vi "medir temp.vi"(2 "multimetro":u16(ring) items=["3458", "34420", "34401"], 3 "Medir Temperatura":bool, 4 "address string":string) -> (1 "Numeric":ext)   [LabVIEW 2014]
uses:
  <vilib>/Analysis/NI_AALBase.lvlib
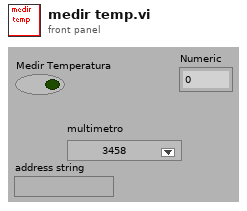
[diagram p1: front panel]
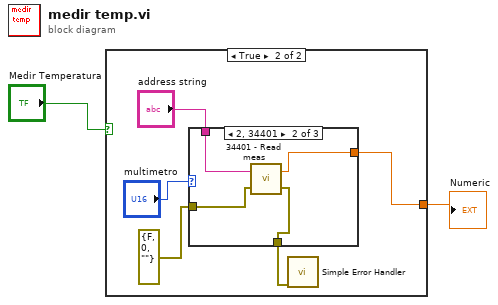
[diagram p0: block diagram]
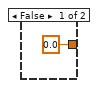
[diagram p2: hidden frame]
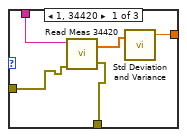
[diagram p3: hidden frame]
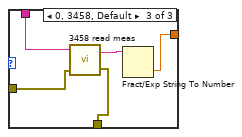
[diagram p4: hidden frame]
diagram:
  n1 = case shown="True" "Medir Temperatura" {
    tunnel: [0.0 ("mean") w4] -> w2
    frame False {
    }
    frame True {
      n2 = case shown="2, 34401" "multimetro" {
        tunnel: "address string" -> [w10 w16 w22]
        tunnel: errorcluster {"status"=FALSE, "code"=0, "source"=""} ("error in (no error)") -> [w11 w17 w21]
        tunnel: [w12 w14 w20] -> w5
        tunnel: [w13 w15 w19] -> w4
        frame 1, 34420 {
          n3 = call "Read Meas 34420.vi"("address string"=w10, "error in (no error)"=w11) -> ("Measurement"=w9:dbl[], "error out"=w12:errorcluster)  [unwired: 3 in]
          n4 = call <vilib>:"Std Deviation and Variance.vi"("X"=w9) -> ("mean"=w13:dbl)  [unwired: 1 in, 2 out]
        }
        frame 2, 34401 {
          n5 = call "34401 - Read meas.vi"("error in (no error)"=w17, "address string"=w16) -> ("error out"=w14:errorcluster, "number"=w15:dbl)
        }
        frame 0, 3458, Default {
          n6 = call "3458 read meas .vi"("error in"=w21, "address string"=w22) -> ("error out"=w20:errorcluster, "data"=w18:string)  [unwired: 1 in]
          n7 = Fract/Exp String To Number(string=w18) -> (number=w19:dbl)  [unwired: 3 in, 1 out]
        }
      }
      n8 = call <vilib>:"Simple Error Handler.vi"("error in (no error)"=w5) -> ()  [unwired: 4 in, 5 out]
    }
  }
  "Numeric" <- w2
